vi "Write I.vi"(8 "error in (no error)":errorcluster, 10 "I":dbl[](array[numeric]), 11 "IV_data in":refnum<class "IV_data.lvclass">) -> (0 "error out":errorcluster, 3 "IV_data out":refnum<class "IV_data.lvclass">)   [LabVIEW 2014, in "IV_data.lvclass"]
uses:
  IV_data.lvclass
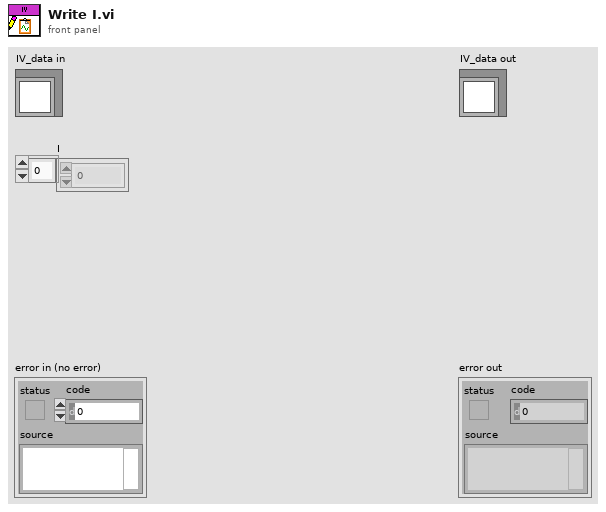
[diagram p1: front panel]
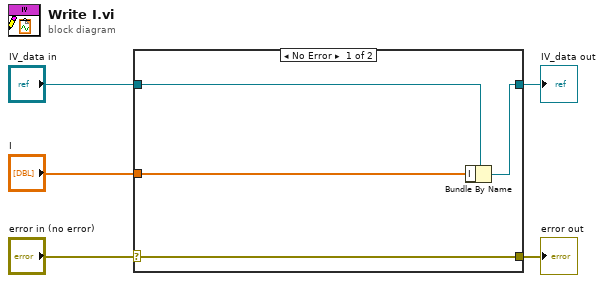
[diagram p0: block diagram]
diagram:
  n1 = case shown="No Error" "error in (no error)" {
    selector: "error in (no error)" -> [w9 w10]
    tunnel: [w9 w10] -> w4
    tunnel: [w7 w11] -> w2
    tunnel: "IV_data in" -> [w8 w11]
    tunnel: "I" -> [w6 _]
    frame No Error {
      n2 = Bundle By Name(cluster=w8, "I"=w6) -> (w7:refnum<class "IV_data.lvclass">)
    }
    frame Error {
    }
  }
  "error out" <- w4
  "IV_data out" <- w2
